vi "FitCurveSelect.vi"() -> ()   [LabVIEW 2016]
uses:
  <vilib>/Analysis/1siggen.llb/Ramp Pattern by Samples.vi
  <vilib>/gmath/NumericalOptimization/Nonlinear Curve Fit LM.vi
  <vilib>/gmath/NI_Gmath.lvlib
  <vilib>/Analysis/NI_AALBase.lvlib
panel:
  out "BestFit":cluster{"Name":string, "Parameter":dbl}[](array[cluster]) caption="Parameter Name          best Fit"
  in  "Guess":T1(array[cluster])=[{"Name"="Offset", "Value"=0.0, "Fit?"=TRUE}, {"Name"="Amplitude", "Value"=3.0, "Fit?"=TRUE}, {"Name"="Time Constant", "Value"=0.5, "Fit?"=TRUE}] caption="Parameter Name          Parameter Guess           Fit?"
  in  "Noise":dbl=0.02
  in  "Simulation parameters":dbl[](array[numeric])=[0.2, 3.0, 0.3] caption="Offset\n\nAmplitude\n\nTime constant"
  out "error out":errorcluster
  in  "stop":bool
  out "XY Graph":cluster{cdb[]}[](graph)
  # "This demo simulates noisy data\nReplace with your experimental data!"
  # "- Run VI\n- Change simulation parameters\n- Change Noise\n- Change Guess\n- enable or disable fitting for some\n   parameters\n\n- Watch the quality of the fit."
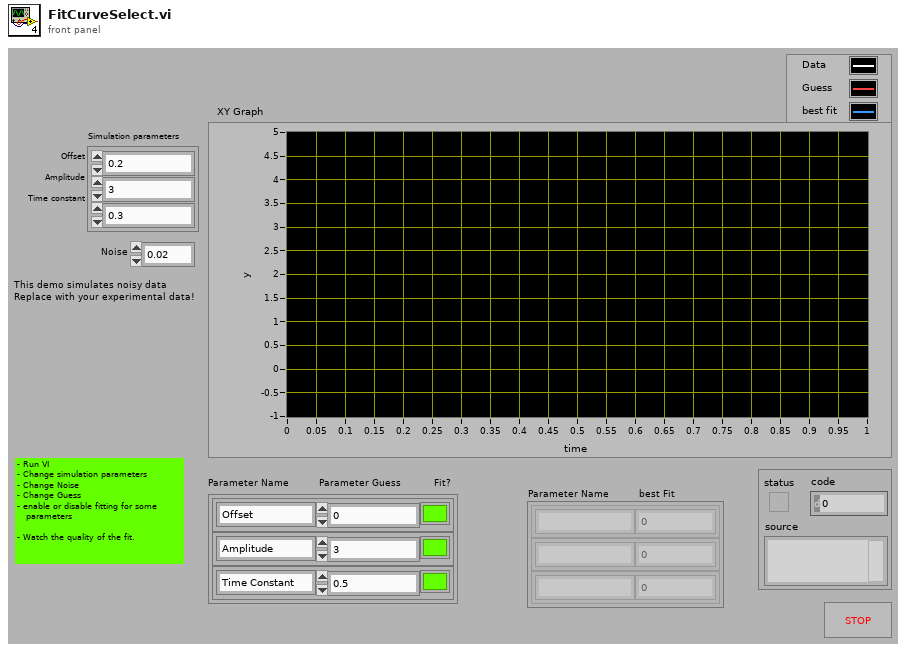
[diagram p1: front panel]
types:
  T1 = cluster{"Name":string, "Value":dbl, "Fit?":bool}[]
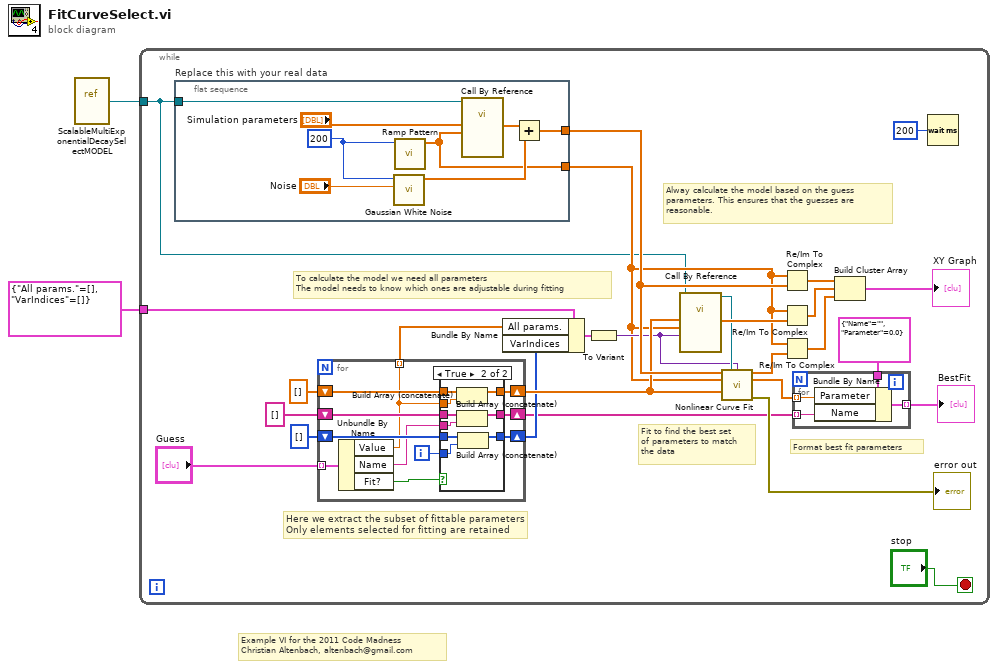
[diagram p0: block diagram]
diagram:
  # "Example VI for the 2011 Code Madness\nChristian Altenbach, altenbach@gmail.com"
  n1 = vi-ref "ScalableMultiExponentialDecaySelectMODEL.vi"() -> (w2:refnum<vi>)
  n2 = while {
    tunnel: w2 -> [w4]
    tunnel: cluster{"All params.":dbl[], "VarIndices":i32[]} {"All params."=[], "VarIndices"=[]} -> [w3]
    stop <- "stop" stop-if-true
    # "Fit to find the best set\nof parameters to match\nthe data"
    # "Format best fit parameters"
    # "Alway calculate the model based on the guess\nparameters. This ensures that the guesses are\nreasonable."
    # "To calculate the model we need all parameters\nThe model needs to know which ones are adjustable during fitting"
    # "Here we extract the subset of fittable parameters\nOnly elements selected for fitting are retained"
    n3 = flat-sequence "Replace this with your real data" {
      tunnel: [w33] -> w19
      tunnel: [w31] -> w5
      tunnel: w4 -> [w30]
      frame #0 {
        w37 = 200 ("samples")
        n4 = call <vilib>:"Gaussian White Noise.vi"("standard deviation"="Noise", "samples"=w37) -> ("Gaussian noise pattern"=w35:dbl[])  [unwired: 8 in, 1 out]
        n5 = call-poly <vilib>:"Ramp Pattern.vi"("samples"=w37) -> ("Ramp Pattern"=w31:dbl[])  [unwired: 9 in, 1 out]
        n6 = call-by-ref "?"(reference=w30, "frequency"=w31, "tau"="Simulation parameters") -> ("Phase"=w36:dbl[])  [unwired: 3 in, 4 out]
        n7 = Add(x=w36, y=w35) -> (x+y=w33:dbl[])
      }
    }
    n8 = for {
      shift-right: [w52] -> w17
      shift-left: dbl[] [] -> [w51]
      tunnel: "Guess" -> [w50] mode=indexing
      tunnel: [w43] -> w14 mode=indexing
      shift-right: [w48] -> w13
      shift-left: i32[] [] -> [w47]
      shift-right: [w44] -> w9
      shift-left: string[] [] -> [w45]
      i -> [w46]
      n9 = Unbundle By Name(w50) -> ("Value"=w43:dbl, "Name"=w42:string, "Fit?"=w49:bool)
      n10 = case shown="True" w49 {
        tunnel: [w55 w63] -> w52
        tunnel: w51 -> [w55 w64]
        tunnel: w43 -> [_ w62]
        tunnel: [w54 w61] -> w48
        tunnel: w47 -> [w54 w60]
        tunnel: w46 -> [_ w59]
        tunnel: [w53 w57] -> w44
        tunnel: w45 -> [w53 w58]
        tunnel: w42 -> [_ w56]
        frame False {
        }
        frame True {
          n11 = Build Array (concatenate)(w64, w62) -> (w63:dbl[])
          n12 = Build Array (concatenate)(w58, w56) -> (w57:string[])
          n13 = Build Array (concatenate)(w60, w59) -> (w61:i32[])
        }
      }
    }
    n14 = Bundle By Name(cluster=w3, "All params."=w14, "VarIndices"=w13) -> (w18:cluster{"All params.":dbl[], "VarIndices":i32[]})
    n15 = To Variant(anything=w18) -> (Variant=w11:variant)
    n16 = call-by-ref "?"(reference=w4, "data"=w11, "frequency"=w5, "tau"=w17) -> (reference out=w22:refnum<vi>, "Phase"=w24:dbl[])  [unwired: 2 in, 3 out]
    n17 = call-poly <vilib>:"Nonlinear Curve Fit.vi"("Y"=w19, "f(x,a)"=w22, "data"=w11, "X"=w5, "initial parameters"=w17) -> ("best nonlinear fit"=w27:dbl[], "best fit parameters"=w8:dbl[], "error out"=→"error out":errorcluster)  [unwired: 5 in, 3 out]
    n18 = Re/Im To Complex(1:w19, 2:w5) -> (0:w29:cdb[])
    n19 = Re/Im To Complex(1:w24, 2:w5) -> (0:w26:cdb[])
    n20 = Re/Im To Complex(1:w27, 2:w5) -> (0:w25:cdb[])
    n21 = for {
      tunnel: w9 -> [w39] mode=indexing
      tunnel: w8 -> [w41] mode=indexing
      tunnel: cluster{"Name":string, "Parameter":dbl} {"Name"="", "Parameter"=0.0} -> [w40]
      tunnel: [w38] -> w6 mode=indexing
      n22 = Bundle By Name(cluster=w40, "Parameter"=w41, "Name"=w39) -> (w38:cluster{"Name":string, "Parameter":dbl})
    }
    "BestFit" <- w6
    n23 = Build Cluster Array(w29, w26, w25) -> (→"XY Graph":cluster{cdb[]}[])
    n24 = Wait (ms)(milliseconds to wait=u32 200) -> ()  [unwired: 1 out]
  }
